vi "Write NCh 1Samp (I32).vi"(5 "timestamp":timestamp, 7 "index_channel":u32, 8 "error in":errorcluster, 9 "data":i32[](array[numeric]), 10 "channels":u32[](array[numeric]), 11 "writer":u64) -> (0 "error out":errorcluster, 3 "writer out":u64)   [LabVIEW 2026, in "synnax_clib.lvlib"]
uses:
  synnax_clib.lvlib
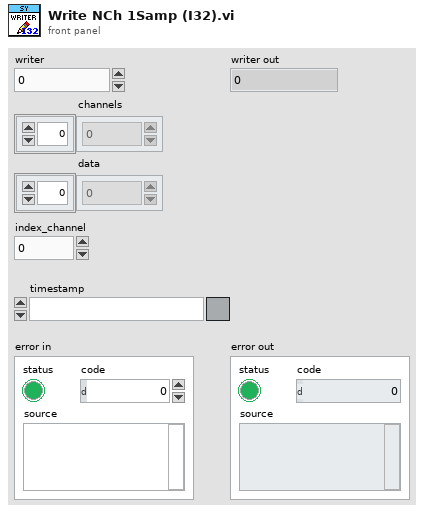
[diagram p1: front panel]
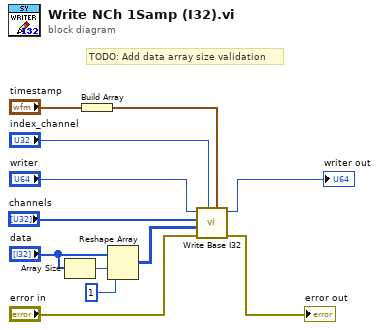
[diagram p0: block diagram]
diagram:
  # "TODO: Add data array size validation"
  n1 = Array Size(array="data") -> (size(s)=w2:i32)
  n2 = Build Array("timestamp") -> (w6:timestamp[])
  n3 = Reshape Array("data", w2, 1) -> (w4:i32[][])
  n4 = call "Write Base I32.vi"("timestamps"=w6, "index_channel"="index_channel", "error in"="error in", "data"=w4, "channels"="channels", "writer"="writer") -> ("error out"=→"error out":errorcluster, "writer out"=→"writer out":u64)  [unwired: 4 in]
